vi "Seconds to time.vi"(11 "Time in Seconds":dbl) -> (1 "Seconds":dbl, 2 "Mins":dbl, 3 "Hours":dbl)   [LabVIEW 2018]
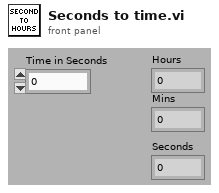
[diagram p1: front panel]
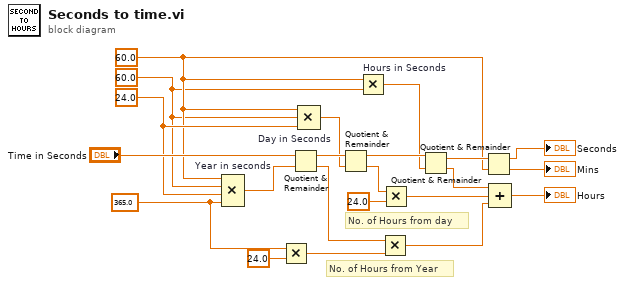
[diagram p0: block diagram]
diagram:
  w3 = 365.0
  w15 = 24.0
  w5 = 60.0
  w6 = 60.0
  # "No. of Hours from day"
  # "No. of Hours from Year"
  n1 = Compound Arithmetic op=MULTIPLY "Year in seconds"(w6, w5, w15, w3) -> (w21:dbl)
  n2 = Multiply(x=w3, y=24.0) -> (x*y=w1:dbl)
  n3 = Quotient & Remainder(x="Time in Seconds", y=w21) -> (x-y*floor(x/y)=w20:dbl, floor(x/y)=w17:dbl)
  n4 = Compound Arithmetic op=MULTIPLY "Day in Seconds"(w6, w5, w15) -> (w16:dbl)
  n5 = Quotient & Remainder(x=w20, y=w16) -> (x-y*floor(x/y)=w19:dbl, floor(x/y)=w14:dbl)
  n6 = Multiply "Hours in Seconds"(x=w6, y=w5) -> (x*y=w18:dbl)
  n7 = Multiply(x=w17, y=w1) -> (x*y=w10:dbl)
  n8 = Multiply(x=w14, y=24.0) -> (x*y=w11:dbl)
  n9 = Quotient & Remainder(x=w19, y=w18) -> (x-y*floor(x/y)=w13:dbl, floor(x/y)=w12:dbl)
  n10 = Quotient & Remainder(x=w13, y=w6) -> (x-y*floor(x/y)=→"Seconds":dbl, floor(x/y)=→"Mins":dbl)
  n11 = Compound Arithmetic op=ADD(w12, w11, w10) -> (→"Hours":dbl)
